vi "ExitAllResource.vi"(8 "error in (no error)":errorcluster) -> (0 "error out":errorcluster)   [LabVIEW 2017]
uses:
  ComVIS/Process/ProcessClass.lvclass
  HardWare/ADLINK/IO/Adlink IO/Adlink IO.lvlib
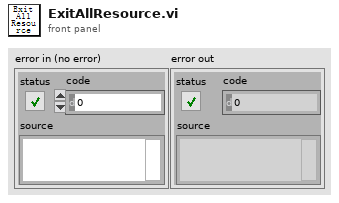
[diagram p1: front panel]
types:
  T1 = typedef "HD Config.ctl" = cluster{" PC":cluster{"PC Address":u8[], "PC Port":i32}, "FCO":cluster{"COM":refnum<visa-resource-name>, "Baudrate":u32}, "DC Power ":cluster{"COM":refnum<visa-resource-name>, "Baudrate":u32}, "PW3336":cluster{"COM":refnum<visa-resource-name>, "Baudrate":u32}, "Lefoo":cluster{"COM":refnum<visa-resource-name>, "Baudrate":u32}, "Tempt&Hum":cluster{"COM":refnum<visa-resource-name>, "Baudrate":u32}, "DIPC":cluster{"COM":refnum<visa-resource-name>}, "Daemon":cluster{"IP Address":string, "Port":u16, "Retry":u16}, "NFC_Cmd":cluster{"COM":refnum<visa-resource-name>, "Baudrate":u32}, "Fail_resume_mode":bool, "GRR":bool, "NFC _Serial":cluster{"COM":refnum<visa-resource-name>, "Baudrate":u32}}
  T2 = cluster{"DI dev":i32[], "DI line":i32[], "Port":i32[], "DO dev":i32[], "DO line":i32[], "IO Data":string[][], "IO f":i16[]}
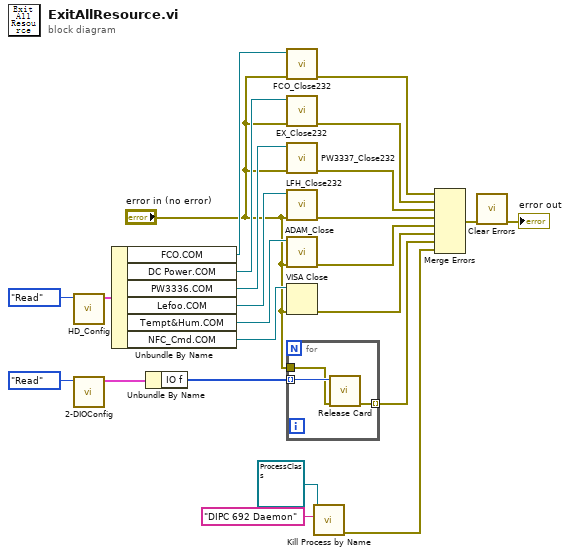
[diagram p0: block diagram]
diagram:
  n1 = call "HD_Config.vi"("Step"=enum16{"Initial", "Write", "Read"}."Read") -> ("HD Config out"=w17:T1)  [unwired: 9 in, 1 out]
  n2 = call "2-DIOConfig.vi"("Step"=enum16{"Initial", "Write", "Read"}."Read") -> ("DIO pra out"=w21:T2)  [unwired: 9 in, 1 out]
  n3 = Unbundle By Name(w17) -> ("FCO.COM"=w16:refnum<visa-resource-name>, "DC Power.COM"=w14:refnum<visa-resource-name>, "PW3336.COM"=w15:refnum<visa-resource-name>, "Lefoo.COM"=w13:refnum<visa-resource-name>, "Tempt&Hum.COM"=w12:refnum<visa-resource-name>, "NFC_Cmd.COM"=w6:refnum<visa-resource-name>)
  n4 = Unbundle By Name(w21) -> ("IO f"=w20:i16[])
  n5 = call "FCO_Close232.vi"("error in (no error)"="error in (no error)", "VISA resource name"=w16) -> ("error out"=w7:errorcluster)  [unwired: 9 in]
  n6 = call "EX_Close232.vi"("error in (no error)"="error in (no error)", "VISA resource name"=w14) -> ("error out"=w8:errorcluster)  [unwired: 9 in]
  n7 = call "PW3337_Close232.vi"("error in (no error)"="error in (no error)", "VISA resource name"=w15) -> ("error out"=w9:errorcluster)  [unwired: 9 in]
  n8 = call "LFH_Close232.vi"("error in (no error)"="error in (no error)", "VISA resource name"=w13) -> ("error out"=w10:errorcluster)  [unwired: 9 in]
  n9 = call "ADAM_Close.vi"("error in (no error)"="error in (no error)", "VISA resource name"=w12) -> ("error out"=w11:errorcluster)  [unwired: 9 in]
  n10 = VISA Close(VISA resource name=w6, error in (no error)="error in (no error)") -> (error out=w5:errorcluster)
  n11 = for {
    tunnel: w20 -> [w27] mode=indexing
    tunnel: [w25] -> w18 mode=indexing
    tunnel: "error in (no error)" -> [w26]
    n12 = call "Release Card.vi"("error in (no error)"=w26, "CardNumber"=w27) -> ("error out"=w25:errorcluster)  [unwired: 8 in, 1 out]
  }
  n13 = call "Kill Process by Name.vi"("processName"="DIPC 692 Daemon", "ProcessClass 输入"=refnum<class "ProcessClass.lvclass"> refnum) -> ("error out"=w3:errorcluster)  [unwired: 8 in, 1 out]
  n14 = Merge Errors(w7, w8, w9, w10, w11, w5, w18, w3) -> (w23:errorcluster)
  n15 = call <vilib>:"Clear Errors.vi"("error in (no error)"=w23) -> ("error out"=→"error out":errorcluster)  [unwired: 5 in, 1 out]
